vi "Write Settings.vi"(0 "class data in":refnum<class "MB_ENGINE.lvclass">, 5 "cluster":T1, 11 "error in (no error)":errorcluster) -> (4 "class data out":refnum<class "MB_ENGINE.lvclass">, 15 "error out":errorcluster)   [LabVIEW 2019, in "MB_ENGINE.lvclass"]
uses:
  MB_ENGINE.lvclass
  Settings.ctl
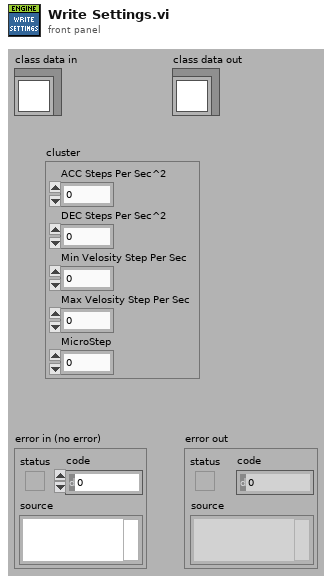
[diagram p1: front panel]
types:
  T1 = typedef "MB_ENGINE.lvclass/Settings.ctl" = cluster{"ACC Steps Per Sec^2":u16, "DEC Steps Per Sec^2":u16, "Min Velosity Step Per Sec":u16, "Max Velosity Step Per Sec":u16, "MicroStep":u16}
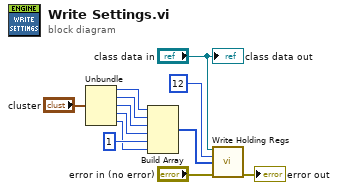
[diagram p0: block diagram]
diagram:
  n1 = Unbundle("cluster") -> ("ACC Steps Per Sec^2"=w10:u16, "DEC Steps Per Sec^2"=w9:u16, "Min Velosity Step Per Sec"=w8:u16, "Max Velosity Step Per Sec"=w7:u16, "MicroStep"=w1:u16)
  n2 = Build Array(w10, w9, w8, w7, u16 1 ("element"), w1) -> (w6:u16[])
  n3 = call-dynamic "Write Holding Regs.vi"("reference in"="class data in", "starting address"=u16 12, "Regs"=w6, "error in (no error)"="error in (no error)") -> ("error out"=→"error out":errorcluster)  [unwired: 11 in]
  "class data out" <- "class data in"
